vi "Pagina login.vi"() -> (0 "pagina out":i16=255, 3 "Nome prodotto selezionato":string)   [LabVIEW 2022 SP3]
uses:
  Labview/Globali.vi
panel:
  out "s_verniciato":bool
  in  "Verniciato":bool caption="PREMERE SE IL GRUPPO E' VERNICIATO"
  out "Foto asse":picture
  in  "Amministratore":bool
  in  "Password":i16(ring) items=["PASSWORD", "01895210", "01946110", "01910410", "10209200"]
  in  "Autocontrollo":i16(ring) items=["AUTOCONTROLLO", "77", "74", "76", "Manfroi"]
  in  "OPERATORE":i16(ring) items=["OPERATORE", "Di Narda Andrea", "Giovannini Gianluca", "Ragona Patrick", "Manfroi Manuel"]
  out "AUTOCONTROLLO":string
  out "Testo allarmi":string caption="ALLARMI"
  out "Testo fase collaudo":string caption="FASE COLLAUDO"
  out "Testo segnalazioni":string caption="SEGNALAZIONI"
  out "Testo messaggi":string caption="MESSAGGI"
  in  "Prova":bool
  out "Login":bool
  in  "stop":bool
  in  "Comandi manuali":bool
  out "Linea":string="CENTAURO"
  out "Picture":picture
  out "Versione SW":dbl=1.0 format="%.2f"
  out "Tipo pagina":string
  in  "MATRICOLA":string
  in  "6. 0":i16(ring) items=["TIPO", "PRODUZIONE", "RICAMBIO", "REVISIONE"]
  in  "Case Constant\n(See Context Help)":bool
  out "Tipo Specifica":i32(ring) items=["", "RP3000", "RP3000", "RP3000", "AAT_2", "AAT_2", "AAT_1_3_4", "AAT_1_3_4", "AAT_1_3_4", "AAT_1_3_4", "AAT_1_3_4", "AAT_1_3_4"]
  in  "4. 0":i16(ring) items=["PRODOTTO", "RP3000 - 60154632", "RP3000 - 60195812", "RP3000 - 504055662", "AAT3000 2° - 60159655", "AAT3000 2° - 60159656", "AAT3000 1° - 60159650", "AAT3000 1° - 60159649", "AAT3000 3° - 60159652", "AAT3000 3° - 60159653", "AAT3000 4° - 60159650", "AAT3000 4° - 60159649"]
  out "Collaudo in corso":string
  out "Messaggio":string caption="Collaudo in corso"
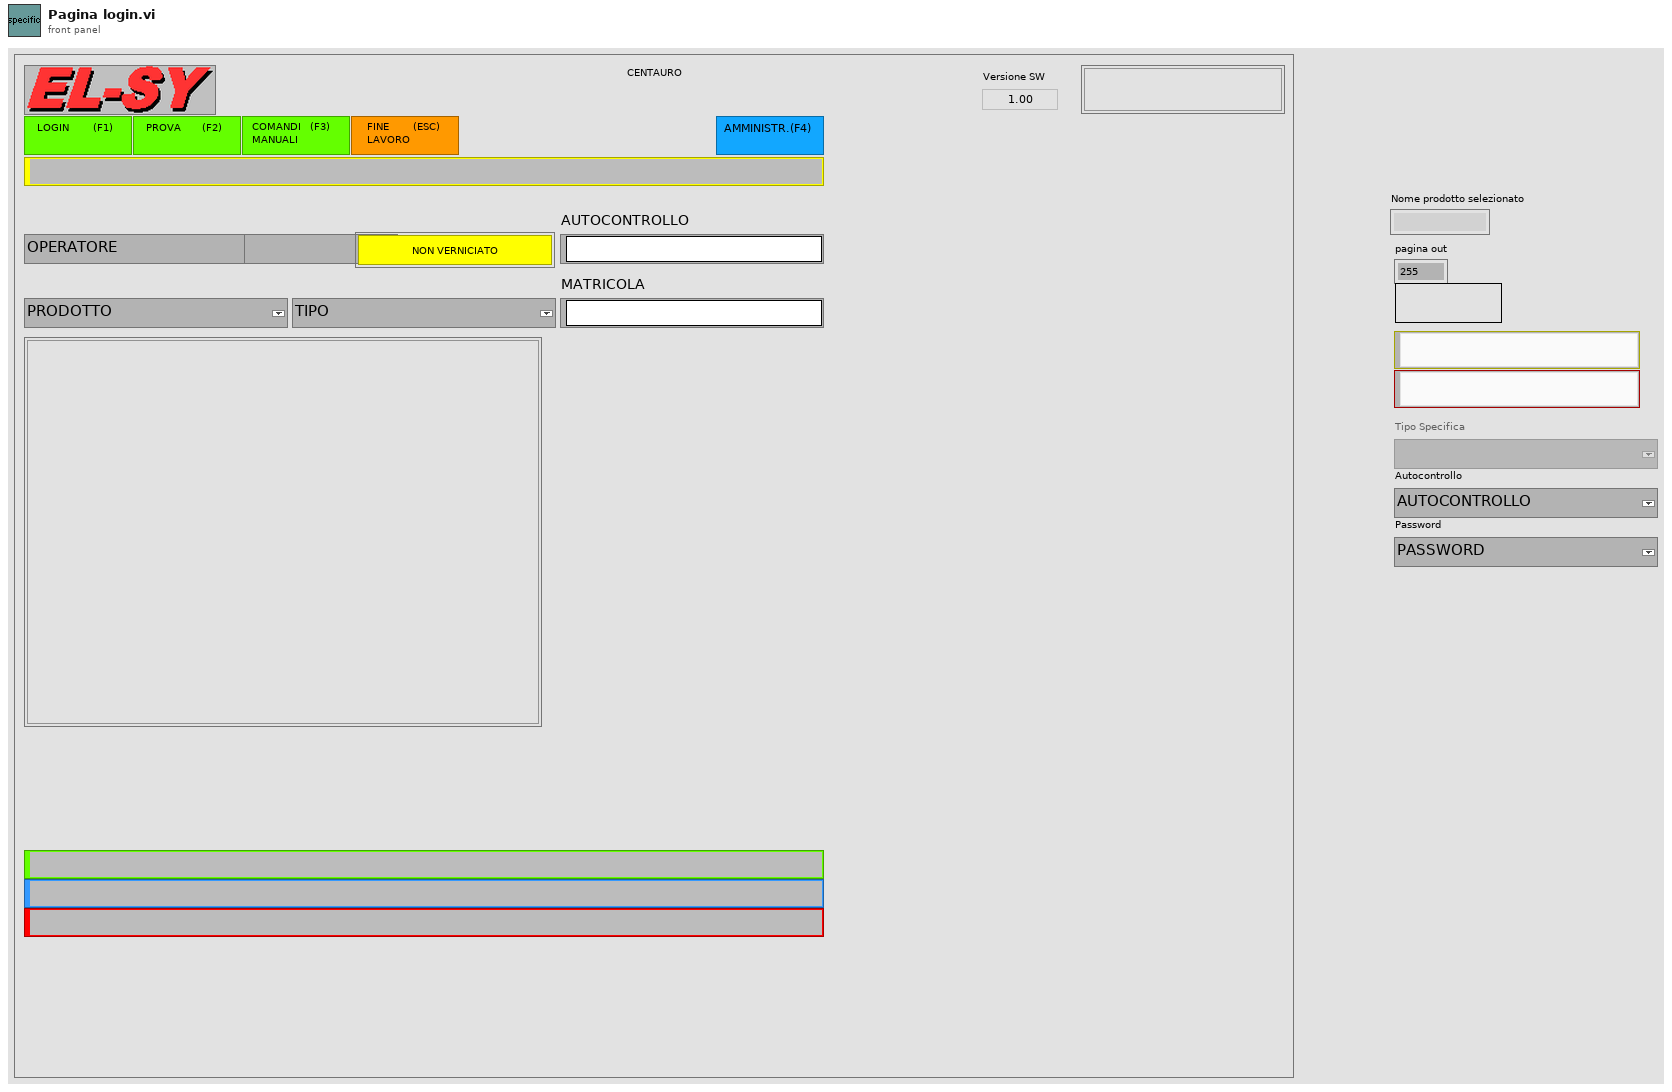
[diagram p1: front panel]
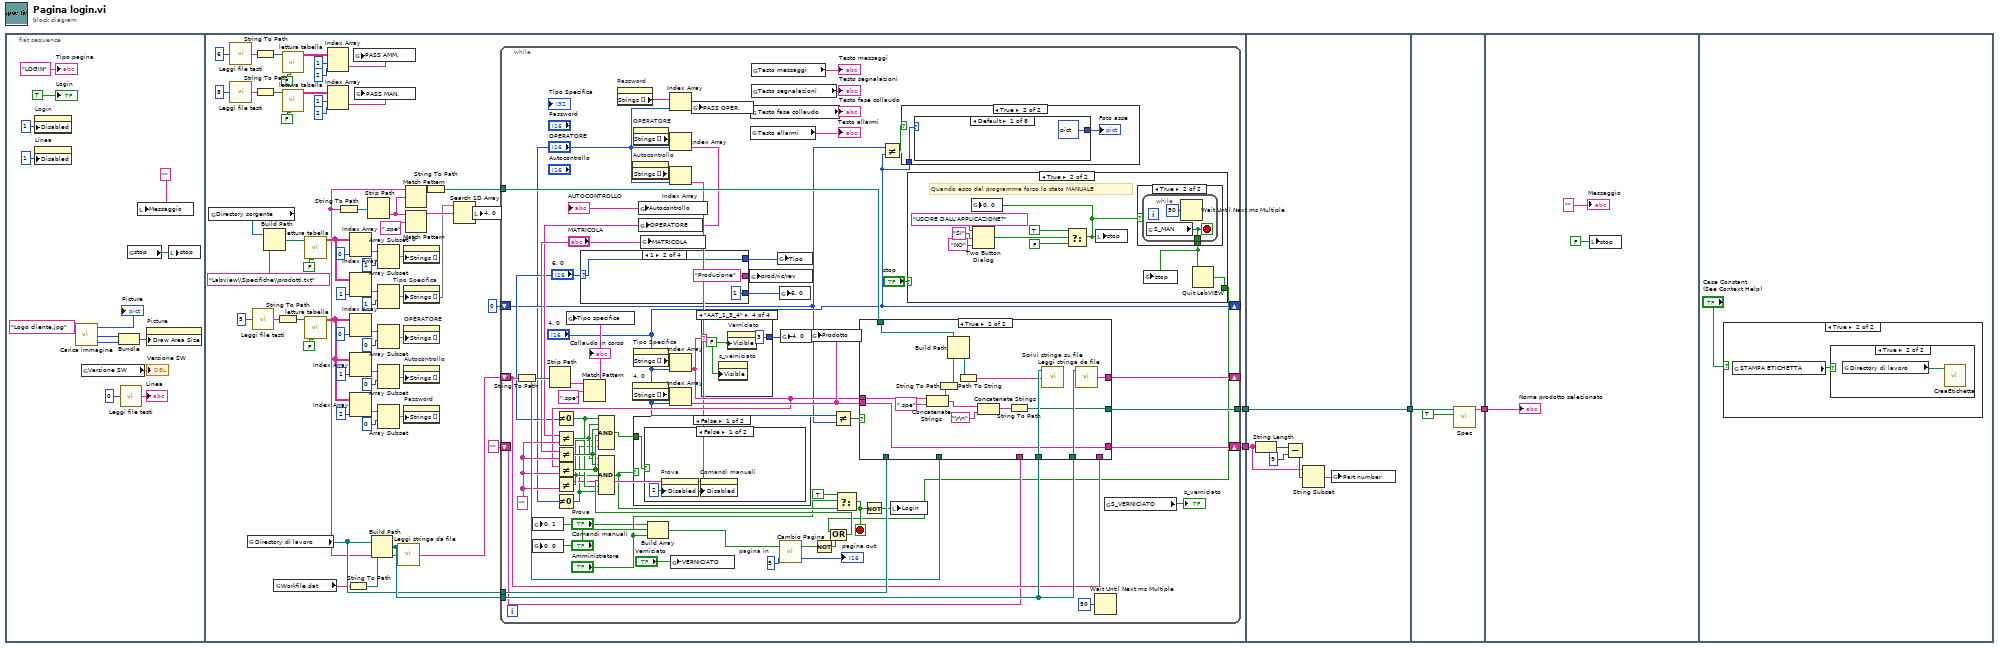
[diagram p0: block diagram]
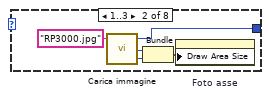
[diagram p3: hidden frame]
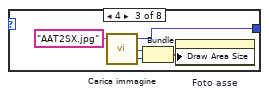
[diagram p4: hidden frame]
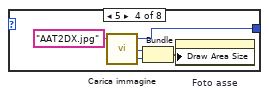
[diagram p5: hidden frame]
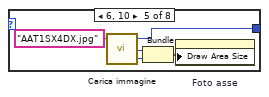
[diagram p6: hidden frame]
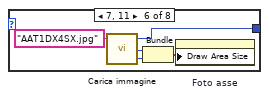
[diagram p7: hidden frame]
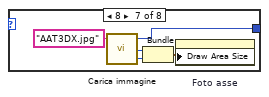
[diagram p8: hidden frame]
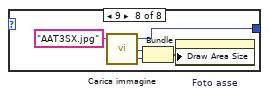
[diagram p9: hidden frame]
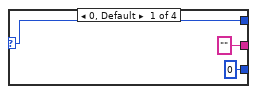
[diagram p10: hidden frame]
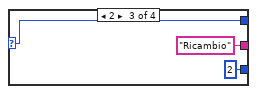
[diagram p11: hidden frame]
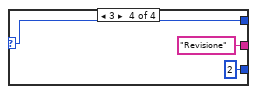
[diagram p12: hidden frame]
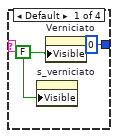
[diagram p13: hidden frame]
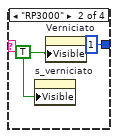
[diagram p14: hidden frame]
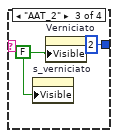
[diagram p15: hidden frame]
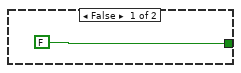
[diagram p16: hidden frame]
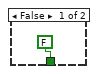
[diagram p17: hidden frame]
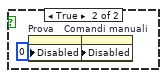
[diagram p18: hidden frame]
diagram:
  n1 = flat-sequence {
    tunnel: [w76] -> w4
    tunnel: [w75] -> w1
    tunnel: w4 -> [w240]
    tunnel: [w240] -> w3
    tunnel: w1 -> [w236]
    tunnel: w3 -> [w242]
    tunnel: [w241] -> w2
    tunnel: w2 -> [w246]
    frame #0 {
      n2 = property on="Login" class="Bool"("Disabled"=u8 1) -> ()  [unwired: 2 in, 2 out]
      n3 = property on="Linea" class="Str"("Disabled"=u8 1) -> ()  [unwired: 2 in, 2 out]
      n4 = call "Carica immagine.vi"("Immagine JPG"="Logo cliente.jpg") -> ("altezza"=w14:i16, "larghezza"=w13:i16, "Picture"=→"Picture":picture)  [unwired: 2 in]
      n5 = global read "Globali.vi" "Versione SW"() -> (→"Versione SW":dbl)
      n6 = Bundle("larghezza"=w13, "altezza"=w14) -> (w15:cluster{"larghezza":i16, "altezza":i16})  [unwired: 1 in]
      n7 = call "Leggi file testi.vi"("Numero riga"=0) -> ("Testo"=→"Linea":string)  [unwired: 3 in, 1 out]
      n8 = global read "Globali.vi" "stop"() -> (w17:bool)
      n9 = local write "Messaggio"("" ("Errore conn. centralina")) -> ()
      n10 = property on="Picture" class="Pict"("Draw Area Size"=w15) -> ()  [unwired: 2 in, 2 out]
      n11 = local write "stop"(w17) -> ()
      "Tipo pagina" <- "LOGIN" ("Tipo pagina")
      "Login" <- TRUE ("Login")
    }
    frame #1 {
      n12 = global read "Globali.vi" "Directory sorgente"() -> (w43:path)
      n13 = call "Leggi file testi.vi"("Numero riga"=6) -> ("Testo"=w33:string)  [unwired: 3 in, 1 out]
      n14 = call "Leggi file testi.vi"("Numero riga"=8) -> ("Testo"=w20:string)  [unwired: 3 in, 1 out]
      n15 = global read "Globali.vi" "Directory di lavoro"() -> (w78:path)
      n16 = call "Leggi file testi.vi"("Numero riga"=5) -> ("Testo"=w36:string)  [unwired: 3 in, 1 out]
      n17 = String To Path(string=w33) -> (path=w34:path)
      n18 = String To Path(string=w20) -> (path=w19:path)
      n19 = Build Path(base path=w43, name or relative path="Labview\\Specifiche\\prodotti.txt") -> (appended path=w54:path)
      n20 = global read "Globali.vi" "Workfile.dat"() -> (w77:string)
      n21 = String To Path(string=w36) -> (path=w35:path)
      n22 = call "lettura tabella.vi"("transpose (no:F)"=FALSE, "file path (dialog if empty)"=w34) -> ("all rows"=w31:string[][])  [unwired: 5 in, 4 out]
      n23 = call "lettura tabella.vi"("transpose (no:F)"=FALSE, "file path (dialog if empty)"=w19) -> ("all rows"=w22:string[][])  [unwired: 5 in, 4 out]
      n24 = call "lettura tabella.vi"("transpose (no:F)"=FALSE, "file path (dialog if empty)"=w54) -> ("all rows"=w70:string[][])  [unwired: 5 in, 4 out]
      n25 = call "lettura tabella.vi"("transpose (no:F)"=FALSE, "file path (dialog if empty)"=w35) -> ("all rows"=w38:string[][])  [unwired: 5 in, 4 out]
      n26 = Index Array(array=w31, index (row)=1 ("disabled index (row)"), index (col)=2 ("disabled index (col)")) -> (element=w27:string)
      n27 = Index Array(array=w22, index (row)=1 ("disabled index (row)"), index (col)=2 ("disabled index (col)")) -> (element=w26:string)
      n28 = String To Path(string=w77) -> (path=w80:path)
      n29 = Index Array(array=w70, index (col)=0 ("disabled index (col)")) -> (element=w67:string[])  [unwired: 1 in]
      n30 = Index Array(array=w70, index (col)=1 ("disabled index (col)")) -> (element=w72:string[])  [unwired: 1 in]
      n31 = Index Array(array=w38, index (col)=0 ("disabled index (col)")) -> (element=w49:string[])  [unwired: 1 in]
      n32 = Index Array(array=w38, index (col)=1 ("disabled index (col)")) -> (element=w45:string[])  [unwired: 1 in]
      n33 = Index Array(array=w38, index (col)=2 ("disabled index (col)")) -> (element=w42:string[])  [unwired: 1 in]
      n34 = global write "Globali.vi" "PASS AMM."(w27) -> ()
      n35 = global write "Globali.vi" "PASS MAN."(w26) -> ()
      n36 = Build Path(base path=w78, name or relative path=w80) -> (appended path=w79:path)
      n37 = Array Subset(array=w67, index=1) -> (w61:string[])  [unwired: 1 in]
      n38 = Array Subset(array=w72, index=1) -> (w53:string[])  [unwired: 1 in]
      n39 = Array Subset(array=w49, index=0) -> (w51:string[])  [unwired: 1 in]
      n40 = Array Subset(array=w45, index=0) -> (w52:string[])  [unwired: 1 in]
      n41 = Array Subset(array=w42, index=0) -> (w39:string[])  [unwired: 1 in]
      n42 = call "Leggi stringa da file.vi"("file path (dialog if empty)"=w79) -> ("character string"=w59:string)  [unwired: 5 in, 3 out]
      n43 = String To Path(string=w59) -> (path=w64:path)
      n44 = Strip Path(path=w64) -> (name=w58:string)  [unwired: 1 out]
      n45 = property on="4. 0" class="Ring (strict)"("Strings []"=w61) -> ()  [unwired: 2 in, 2 out]
      n46 = property on="Tipo Specifica" class="Ring (strict)"("Strings []"=w53) -> ()  [unwired: 2 in, 2 out]
      n47 = property on="OPERATORE" class="Ring (strict)"("Strings []"=w51) -> ()  [unwired: 2 in, 2 out]
      n48 = property on="Autocontrollo" class="Ring (strict)"("Strings []"=w52) -> ()  [unwired: 2 in, 2 out]
      n49 = property on="Password" class="Ring (strict)"("Strings []"=w39) -> ()  [unwired: 2 in, 2 out]
      n50 = Match Pattern(string=w59, regular expression=w58) -> (before substring=w57:string)  [unwired: 1 in, 3 out]
      n51 = Match Pattern(string=w58, regular expression=".spe") -> (before substring=w62:string)  [unwired: 1 in, 3 out]
      n52 = String To Path(string=w57) -> (path=w56:path)
      n53 = Search 1D Array(1D array=w53, element=w62) -> (index of element=w60:i32)  [unwired: 1 in]
      n54 = local write "4. 0"(w60) -> ()
      n55 = while {
        tunnel: w79 -> [w138]
        shift-right: [w141] -> _
        shift-left: w59 -> [w137]
        tunnel: w78 -> [w140]
        tunnel: [w136] -> w76
        shift-right: [w129] -> w75
        shift-left: "" -> [w128]
        shift-right: ["4. 0"] -> _
        shift-left: 0 ("NOME PRODOTTO") -> [w89]
        tunnel: w56 -> [w125]
        stop <- w94 stop-if-true
        w108 = ""
        w133 = u8 5  # pagina in
        n56 = String To Path(string=w137) -> (path=w135:path)
        n57 = global write "Globali.vi" "0. 1"("Prova") -> ()
        n58 = global write "Globali.vi" "0. 0"("Comandi manuali") -> ()
        n59 = Strip Path(path=w135) -> (name=w139:string)  [unwired: 1 out]
        n60 = Not Equal To 0?(x="6. 0") -> (x != 0?=w109:bool)
        n61 = Not Equal?(x="MATRICOLA", y=w108) -> (x != y?=w118:bool)
        n62 = Not Equal To 0?(x="OPERATORE") -> (x != 0?=w85:bool)
        n63 = case shown="1" "6. 0" {
          selector: "6. 0" -> [w182 w185 w188 w191]
          tunnel: [0 1 2 2] -> w97
          tunnel: ["" ("prod/ric/rev") "Produzione" ("prod/ric/rev") "Ricambio" ("prod/ric/rev") "Revisione" ("prod/ric/rev")] -> w88
          tunnel: [w182 w185 w188 w191] -> w87
          frame 0, Default {
          }
          frame 1 {
          }
          frame 2 {
          }
          frame 3 {
          }
        }
        n64 = Match Pattern(string=w139, regular expression=".spe") -> (before substring=w134:string)  [unwired: 1 in, 3 out]
        "Collaudo in corso" <- w134
        n65 = global write "Globali.vi" "Tipo specifica"(w134) -> ()
        n66 = property on="Password" class="Ring (strict)"() -> ("Strings []"=w99:string[])  [unwired: 2 in, 2 out]
        n67 = property on="Autocontrollo" class="Ring (strict)"() -> ("Strings []"=w102:string[])  [unwired: 2 in, 2 out]
        n68 = property on="4. 0" class="Ring (strict)"() -> ("Strings []"=w123:string[])  [unwired: 2 in, 2 out]
        n69 = property on="OPERATORE" class="Ring (strict)"() -> ("Strings []"=w103:string[])  [unwired: 2 in, 2 out]
        n70 = property on="Tipo Specifica" class="Ring (strict)"() -> ("Strings []"=w122:string[])  [unwired: 2 in, 2 out]
        n71 = global write "Globali.vi" "MATRICOLA"("MATRICOLA") -> ()
        n72 = Build Array("Prova", "Comandi manuali", "Amministratore") -> (w132:bool[])
        n73 = Index Array(array=w99, index="OPERATORE") -> (element=w96:string)
        n74 = Index Array(array=w103, index="OPERATORE") -> (element=w100:string)
        n75 = Not Equal?(x=w100, y=w108) -> (x != y?=w117:bool)
        n76 = global write "Globali.vi" "OPERATORE"(w100) -> ()
        n77 = Index Array(array=w102, index="OPERATORE") -> (element=w101:string)
        "AUTOCONTROLLO" <- w101
        n78 = Not Equal?(x=w101, y=w108) -> (x != y?=w107:bool)
        n79 = global write "Globali.vi" "Autocontrollo"(w101) -> ()
        n80 = Index Array(array=w122, index="4. 0") -> (element=w104:string)
        n81 = Not Equal?(x=w104, y=w108) -> (x != y?=w119:bool)
        n82 = Compound Arithmetic op=AND(w109, w117, w118, w119, w107, w85) -> (w120:bool)
        n83 = Index Array(array=w123, index="4. 0") -> (element=w110:string)
        n84 = global write "Globali.vi" "VERNICIATO"("Verniciato") -> ()
        n85 = global write "Globali.vi" "PASS OPER."(w96) -> ()
        n86 = case shown="\"AAT_1_3_4\"" w104 {
          tunnel: [0 1 2 3] -> w105
          frame Default {
            w194 = FALSE ("Visible")
            n87 = property on="s_verniciato" class="Bool (strict)"("Visible"=w194) -> ()  [unwired: 2 in, 2 out]
            n88 = property on="Verniciato" class="Bool (strict)"("Visible"=w194) -> ()  [unwired: 2 in, 2 out]
          }
          frame "RP3000" {
            w196 = TRUE ("Visible")
            n89 = property on="s_verniciato" class="Bool (strict)"("Visible"=w196) -> ()  [unwired: 2 in, 2 out]
            n90 = property on="Verniciato" class="Bool (strict)"("Visible"=w196) -> ()  [unwired: 2 in, 2 out]
          }
          frame "AAT_2" {
            w198 = FALSE ("Visible")
            n91 = property on="s_verniciato" class="Bool (strict)"("Visible"=w198) -> ()  [unwired: 2 in, 2 out]
            n92 = property on="Verniciato" class="Bool (strict)"("Visible"=w198) -> ()  [unwired: 2 in, 2 out]
          }
          frame "AAT_1_3_4" {
            w200 = FALSE ("Visible")
            n93 = property on="s_verniciato" class="Bool (strict)"("Visible"=w200) -> ()  [unwired: 2 in, 2 out]
            n94 = property on="Verniciato" class="Bool (strict)"("Visible"=w200) -> ()  [unwired: 2 in, 2 out]
          }
        }
        n95 = global write "Globali.vi" "prod/ric/rev"(w88) -> ()
        n96 = global read "Globali.vi" "Testo fase collaudo"() -> (→"Testo fase collaudo":string)
        n97 = global read "Globali.vi" "Testo allarmi"() -> (→"Testo allarmi":string)
        n98 = global read "Globali.vi" "Testo messaggi"() -> (→"Testo messaggi":string)
        n99 = global read "Globali.vi" "Testo segnalazioni"() -> (→"Testo segnalazioni":string)
        n100 = global write "Globali.vi" "Tipo"(w87) -> ()
        n101 = global write "Globali.vi" "6. 0"(w97) -> ()
        n102 = call "Cambio Pagina.vi"("pagina in"=w133, "pulsanti"=w132) -> ("pagina out"=→"pagina out":u8, "premuto"=w131:bool)
        n103 = global write "Globali.vi" "4. 0"(w105) -> ()
        n104 = global write "Globali.vi" "Prodotto"(w110) -> ()
        n105 = Not(x=w131) -> (.not. x?=w130:bool)
        n106 = Not Equal?(x="4. 0", y=w89) -> (x != y?=w127:bool)
        n107 = case shown="True" w127 {
          tunnel: [w220 w232] -> w141
          tunnel: w138 -> [_ w231]
          tunnel: w140 -> [_ _]
          tunnel: w138 -> [_ w230]
          tunnel: w137 -> [w220 _]
          tunnel: [w219 w224] -> w136
          tunnel: w135 -> [w219 _]
          tunnel: [w218 w222] -> w129
          tunnel: w128 -> [w218 _]
          tunnel: w104 -> [_ w223]
          tunnel: w110 -> [_ w222]
          tunnel: w125 -> [_ w221]
          frame False {
          }
          frame True {
            n108 = Concatenate Strings(w223, ".spe" ("string")) -> (w227:string)
            n109 = String To Path(string=w227) -> (path=w229:path)
            n110 = Build Path(base path=w221, name or relative path=w229) -> (appended path=w234:path)
            n111 = Path To String(path=w234) -> (string=w228:string)
            n112 = Concatenate Strings(w227, "\r\n") -> (w225:string)
            n113 = String To Path(string=w225) -> (path=w224:path)
            n114 = call "Scrivi stringa su file.vi"("character string"=w228, "file path (dialog if empty)"=w230) -> ()  [unwired: 3 in, 1 out]
            n115 = call "Leggi stringa da file.vi"("file path (dialog if empty)"=w231) -> ("character string"=w232:string)  [unwired: 5 in, 3 out]
          }
        }
        n116 = Not Equal?(x=w89, y="4. 0") -> (x != y?=w91:bool)
        n117 = case shown="True" w91 {
          tunnel: "4. 0" -> [_ w144]
          frame False {
          }
          frame True {
            n118 = case shown="Default" w144 {
              tunnel: [picture data[5B] ("Picture") w148 w153 w158 w163 w168 w173 w178] -> w145
              frame Default {
              }
              frame 1..3 {
                n119 = call "Carica immagine.vi"("Immagine JPG"="RP3000.jpg") -> ("altezza"=w149:i16, "larghezza"=w150:i16, "Picture"=w148:picture)  [unwired: 2 in]
                n120 = Bundle("larghezza"=w150, "altezza"=w149) -> (w151:cluster{"larghezza":i16, "altezza":i16})  [unwired: 1 in]
                n121 = property on="Foto asse" class="Pict"("Draw Area Size"=w151) -> ()  [unwired: 2 in, 2 out]
              }
              frame 4 {
                n122 = call "Carica immagine.vi"("Immagine JPG"="AAT2SX.jpg") -> ("altezza"=w154:i16, "larghezza"=w155:i16, "Picture"=w153:picture)  [unwired: 2 in]
                n123 = Bundle("larghezza"=w155, "altezza"=w154) -> (w156:cluster{"larghezza":i16, "altezza":i16})  [unwired: 1 in]
                n124 = property on="Foto asse" class="Pict"("Draw Area Size"=w156) -> ()  [unwired: 2 in, 2 out]
              }
              frame 5 {
                n125 = call "Carica immagine.vi"("Immagine JPG"="AAT2DX.jpg") -> ("altezza"=w159:i16, "larghezza"=w160:i16, "Picture"=w158:picture)  [unwired: 2 in]
                n126 = Bundle("larghezza"=w160, "altezza"=w159) -> (w161:cluster{"larghezza":i16, "altezza":i16})  [unwired: 1 in]
                n127 = property on="Foto asse" class="Pict"("Draw Area Size"=w161) -> ()  [unwired: 2 in, 2 out]
              }
              frame 6, 10 {
                n128 = call "Carica immagine.vi"("Immagine JPG"="AAT1SX4DX.jpg") -> ("altezza"=w164:i16, "larghezza"=w165:i16, "Picture"=w163:picture)  [unwired: 2 in]
                n129 = Bundle("larghezza"=w165, "altezza"=w164) -> (w166:cluster{"larghezza":i16, "altezza":i16})  [unwired: 1 in]
                n130 = property on="Foto asse" class="Pict"("Draw Area Size"=w166) -> ()  [unwired: 2 in, 2 out]
              }
              frame 7, 11 {
                n131 = call "Carica immagine.vi"("Immagine JPG"="AAT1DX4SX.jpg") -> ("altezza"=w169:i16, "larghezza"=w170:i16, "Picture"=w168:picture)  [unwired: 2 in]
                n132 = Bundle("larghezza"=w170, "altezza"=w169) -> (w171:cluster{"larghezza":i16, "altezza":i16})  [unwired: 1 in]
                n133 = property on="Foto asse" class="Pict"("Draw Area Size"=w171) -> ()  [unwired: 2 in, 2 out]
              }
              frame 8 {
                n134 = call "Carica immagine.vi"("Immagine JPG"="AAT3DX.jpg") -> ("altezza"=w174:i16, "larghezza"=w175:i16, "Picture"=w173:picture)  [unwired: 2 in]
                n135 = Bundle("larghezza"=w175, "altezza"=w174) -> (w176:cluster{"larghezza":i16, "altezza":i16})  [unwired: 1 in]
                n136 = property on="Foto asse" class="Pict"("Draw Area Size"=w176) -> ()  [unwired: 2 in, 2 out]
              }
              frame 9 {
                n137 = call "Carica immagine.vi"("Immagine JPG"="AAT3SX.jpg") -> ("altezza"=w179:i16, "larghezza"=w180:i16, "Picture"=w178:picture)  [unwired: 2 in]
                n138 = Bundle("larghezza"=w180, "altezza"=w179) -> (w181:cluster{"larghezza":i16, "altezza":i16})  [unwired: 1 in]
                n139 = property on="Foto asse" class="Pict"("Draw Area Size"=w181) -> ()  [unwired: 2 in, 2 out]
              }
            }
            "Foto asse" <- w145
          }
        }
        n140 = case shown="True" "stop" {
          tunnel: [FALSE ("x = y?") w203] -> w83
          frame False {
          }
          frame True {
            # "Quando esco dal programma forzo lo stato MANUALE"
            n141 = Two Button Dialog(message="USCIRE DALL'APPLICAZIONE?" ("T button name (\"OK\")"), 1:"NO" ("F button name (\"Cancel\")"), 2:"SI" ("T button name (\"OK\")")) -> (T button?=w206:bool)
            n142 = Select(t=TRUE, s=w206, f=FALSE) -> (s? t:f=w204:bool)
            n143 = global write "Globali.vi" "0. 0"(w204) -> ()
            n144 = local write "stop"(w204) -> ()
            n145 = case shown="True" w204 {
              tunnel: [FALSE ("S_MAN") w212] -> w203
              frame False {
              }
              frame True {
                n146 = while {
                  tunnel: [w213] -> w212
                  stop <- w213 stop-if-true
                  n147 = global read "Globali.vi" "S_MAN"() -> (w213:bool)
                  n148 = Wait Until Next ms Multiple(millisecond multiple=u32 50) -> ()  [unwired: 1 out]
                }
              }
            }
            n149 = global write "Globali.vi" "stop"(w203) -> ()
            n150 = Quit LabVIEW(quit? (T)=w203) -> ()
          }
        }
        n151 = Compound Arithmetic op=OR(w83, w130) -> (w126:bool)
        n152 = Compound Arithmetic op=AND(w117, w118, w119, w107, w126, w109, w85) -> (w95:bool)
        n153 = case shown="False" w95 {
          tunnel: w120 -> [w215 _]
          frame False {
            n154 = case shown="False" w215 {
              frame False {
                w216 = u8 2 ("Disabled")
                n155 = property on="Prova" class="Bool"("Disabled"=w216) -> ()  [unwired: 2 in, 2 out]
                n156 = property on="Comandi manuali" class="Bool"("Disabled"=w216) -> ()  [unwired: 2 in, 2 out]
              }
              frame True {
                w217 = u8 0 ("Disabled")
                n157 = property on="Prova" class="Bool"("Disabled"=w217) -> ()  [unwired: 2 in, 2 out]
                n158 = property on="Comandi manuali" class="Bool"("Disabled"=w217) -> ()  [unwired: 2 in, 2 out]
              }
            }
          }
          frame True {
          }
        }
        n159 = Select(t=TRUE, s="Amministratore", f=w95) -> (s? t:f=w94:bool)
        n160 = Not(x=w94) -> (.not. x?=w116:bool)
        n161 = local write "Login"(w116) -> ()
        n162 = Wait Until Next ms Multiple(millisecond multiple=u32 50) -> ()  [unwired: 1 out]
        n163 = global read "Globali.vi" "S_VERNICIATO"() -> (→"s_verniciato":bool)
      }
    }
    frame #2 {
      n164 = String Length(string=w236) -> (length=w239:i32)
      n165 = Subtract(x=w239, y=9) -> (x-y=w237:i32)
      n166 = String Subset(string=w236, offset (0)=w237) -> (substring=w235:string)  [unwired: 1 in]
      n167 = global write "Globali.vi" "Part number"(w235) -> ()
    }
    frame #3 {
      n168 = call "Spec.vi"("Carica specifica da programma"=TRUE, "file path"=w242) -> ("Nome prodotto selezionato"=w241:string)  [unwired: 4 in, 1 out]
    }
    frame #4 {
      n169 = local write "stop"(FALSE ("stop")) -> ()
      "Nome prodotto selezionato" <- w246
      "Messaggio" <- "" ("Errore conn. centralina")
    }
    frame #5 {
      n170 = case shown="True" "Case Constant\n(See Context Help)" {
        frame False {
        }
        frame True {
          n171 = global read "Globali.vi" "STAMPA ETICHETTA"() -> (w248:bool)
          n172 = case shown="True" w248 {
            frame False {
            }
            frame True {
              n173 = global read "Globali.vi" "Directory di lavoro"() -> (w249:path)
              n174 = call "CreaEtichetta.vi"("Directory di lavoro"=w249) -> ()  [unwired: 5 in, 4 out]
            }
          }
        }
      }
    }
  }
